vi "Digital Write 1 Channel.vi"(8 "error constant":errorcluster, 9 "Value":bool=TRUE, 10 "Channel":i32, 11 "Arduino.lvclass":refnum<class "Arduino.lvclass">) -> (0 "error IO":errorcluster, 3 "Arduino.lvclass 2":refnum<class "Arduino.lvclass">)   [LabVIEW 2018, in "Arduino.lvclass"]
uses:
  Arduino.lvclass
  <vilib>/MakerHub/LINX/Public/Peripherals/Digital/Digital Write 1 Chan.vi
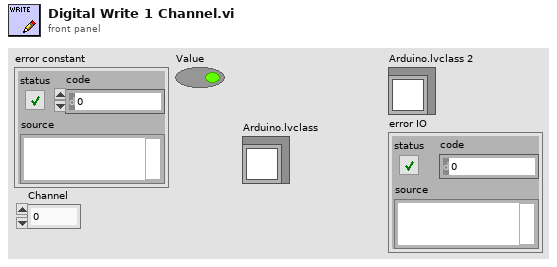
[diagram p1: front panel]
types:
  T1 = typedef "LMH-LINX.lvlib/LINX Ref.ctl" = cluster{"IO":T2, "Interface":T3, "LINX Device Config":T4}
  T2 = typedef "LMH-LINX.lvlib/Platform.ctl" = enum16{"Remote", "Local"}
  T3 = typedef "LMH-LINX.lvlib/Interface.ctl" = enum16{"Serial", "TCP"}
  T4 = typedef "LMH-LINX.lvlib/Device.lvlib/LINX Device Config.ctl" = cluster{"Interface":T3, "COM Port":refnum<visa-resource-name>, "TCP Configuration":T5, "Device Family":u8, "Device ID":u8, "Device Name":string, "TCP Ref":refnum<k5>, "Channels":T6}
  T5 = typedef "LMH-LINX.lvlib/Device.lvlib/TCP Config.ctl" = cluster{"IP Address":string, "Port":u16}
  T6 = typedef "LMH-LINX.lvlib/Channels.ctl" = cluster{"DI":u8[], "DO":u8[], "AI":u8[], "AO":u8[], "PWM":u8[], "QE":u8[], "UART":u8[], "I2C 2":u8[], "SPI":u8[], "CAN":u8[], "Servo":u8[], "AI Ref (V)":dbl, "AI Resolution (Bits)":u8, "AO Ref (V)":dbl, "AO Resolution (Bits)":u8}
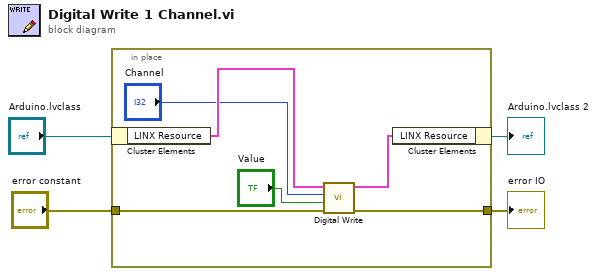
[diagram p0: block diagram]
diagram:
  n1 = in-place {
    in-place-border: "error constant" -> [w6]
    in-place-border: [w5] -> w1
    n2 = in-place-cluster #1("Arduino.lvclass") -> ("LINX Resource"=w10:T1)
    n3 = call-poly <vilib>:"Digital Write.vi"("Error In"=w6, "Output Value"="Value", "DO Channel"="Channel", "LINX Resource"=w10) -> ("Error Out"=w5:errorcluster, "LINX Resource"=w9:T1)  [unwired: 6 in]
    n4 = in-place-cluster #1("LINX Resource"=w9) -> (→"Arduino.lvclass 2":refnum<class "Arduino.lvclass">)
  }
  "error IO" <- w1
